vi "Uncertainty Calcs.vi"(0 "Suction Pressure Random Uncertainty in":dbl, 1 "Suction Temperature Random Uncertainty in":dbl, 5 "Discharge Pressure Random Uncertainty in":dbl, 7 "Systematic Uncertainty of Tsuc":dbl, 9 "Systematic Uncertainty of Psuc":dbl, 12 "Systematic Uncertainty of Pdis":dbl) -> (2 "Suction Pressure Random Uncertainty out":dbl, 3 "Suction Temperature Random Uncertainty out":dbl, 4 "Total Suction Temperature Uncertainty":dbl, 6 "Tsuc Random Contribution to Total":dbl, 8 "Psuc Random Contribution to Total":dbl, 10 "Pdis Random Contribution to Total":dbl, 13 "Discharge Pressure Random Uncertainty out":dbl, 14 "Total Discharge Pressure Uncertainty":dbl, 15 "Total Suction Pressure Uncertainty":dbl)   [LabVIEW 2017]
doc: "This VI calculates the random and total uncertainty of each of the key variables (suction/discharge pressure, suction temperature)."
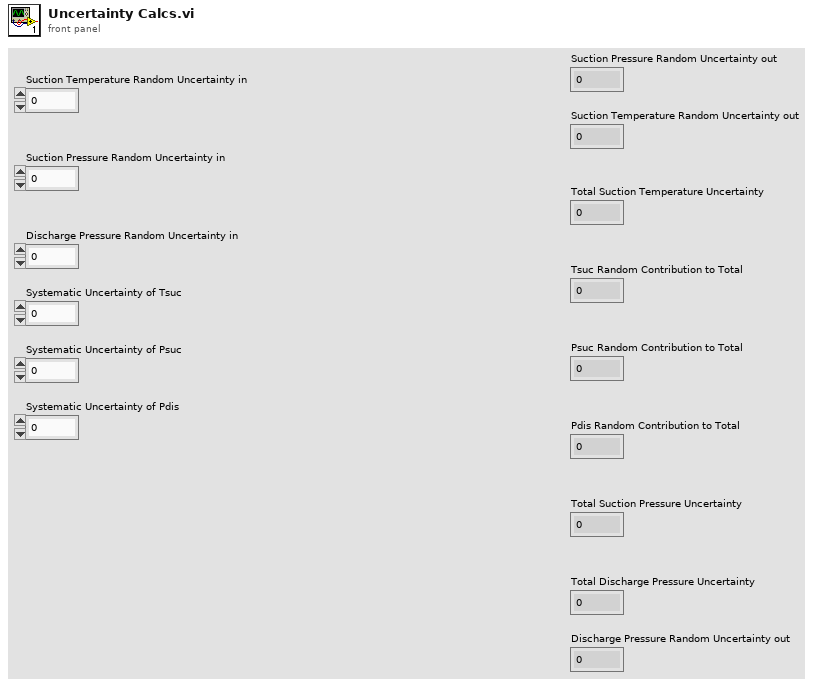
[diagram p1: front panel]
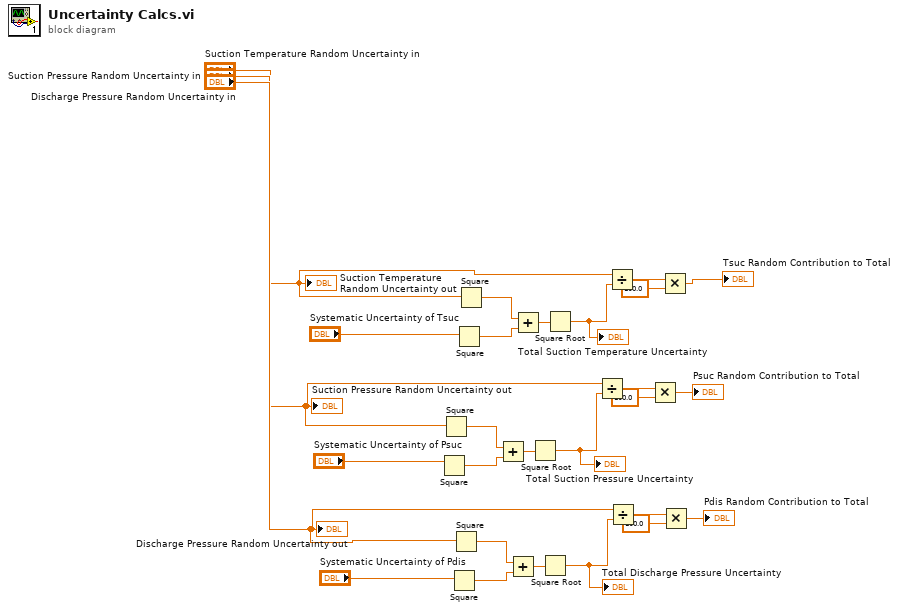
[diagram p0: block diagram]
diagram:
  n1 = Square(x="Systematic Uncertainty of Psuc") -> (x^2=w6:dbl)
  n2 = Square(x="Suction Pressure Random Uncertainty in") -> (x^2=w5:dbl)
  n3 = Square(x="Systematic Uncertainty of Pdis") -> (x^2=w10:dbl)
  n4 = Square(x="Discharge Pressure Random Uncertainty in") -> (x^2=w9:dbl)
  n5 = Square(x="Systematic Uncertainty of Tsuc") -> (x^2=w3:dbl)
  n6 = Square(x="Suction Temperature Random Uncertainty in") -> (x^2=w2:dbl)
  n7 = Add(x=w5, y=w6) -> (x+y=w7:dbl)
  n8 = Add(x=w9, y=w10) -> (x+y=w11:dbl)
  n9 = Add(x=w2, y=w3) -> (x+y=w4:dbl)
  n10 = Square Root(x=w7) -> (sqrt(x)=w20:dbl)
  "Total Suction Pressure Uncertainty" <- w20
  n11 = Square Root(x=w11) -> (sqrt(x)=w25:dbl)
  "Total Discharge Pressure Uncertainty" <- w25
  n12 = Square Root(x=w4) -> (sqrt(x)=w13:dbl)
  "Total Suction Temperature Uncertainty" <- w13
  n13 = Divide(x="Suction Pressure Random Uncertainty in", y=w20) -> (x/y=w18:dbl)
  n14 = Divide(x="Suction Temperature Random Uncertainty in", y=w13) -> (x/y=w15:dbl)
  n15 = Divide(x="Discharge Pressure Random Uncertainty in", y=w25) -> (x/y=w23:dbl)
  n16 = Multiply(x=w18, y=100.0) -> (x*y=→"Psuc Random Contribution to Total":dbl)
  n17 = Multiply(x=w15, y=100.0) -> (x*y=→"Tsuc Random Contribution to Total":dbl)
  n18 = Multiply(x=w23, y=100.0) -> (x*y=→"Pdis Random Contribution to Total":dbl)
  "Suction Temperature Random Uncertainty out" <- "Suction Temperature Random Uncertainty in"
  "Suction Pressure Random Uncertainty out" <- "Suction Pressure Random Uncertainty in"
  "Discharge Pressure Random Uncertainty out" <- "Discharge Pressure Random Uncertainty in"
